vi "GetUIRef.vi"(8 "error in (no error)":errorcluster, 11 "Controller in":refnum<class "Controller.lvclass">) -> (0 "error out":errorcluster, 2 "VIRef":refnum<vi>, 3 "Controller out":refnum<class "Controller.lvclass">)   [LabVIEW 2020, in "UIHome.lvlib" / "Controller.lvclass"]
uses:
  Controller.lvclass
  Controller.lvclass/Controller.ctl
  iView/iView.lvclass
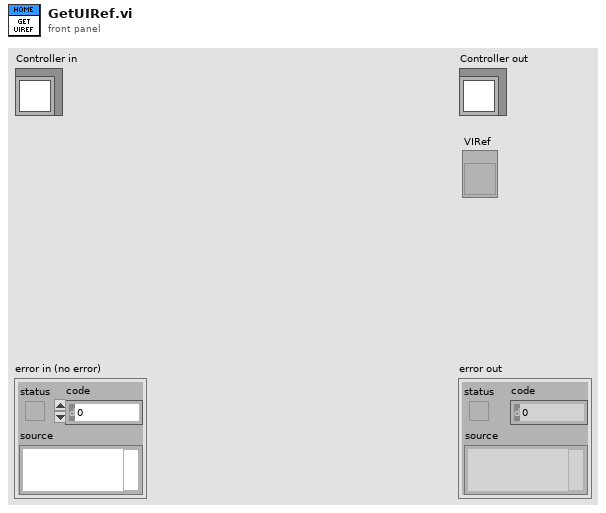
[diagram p1: front panel]
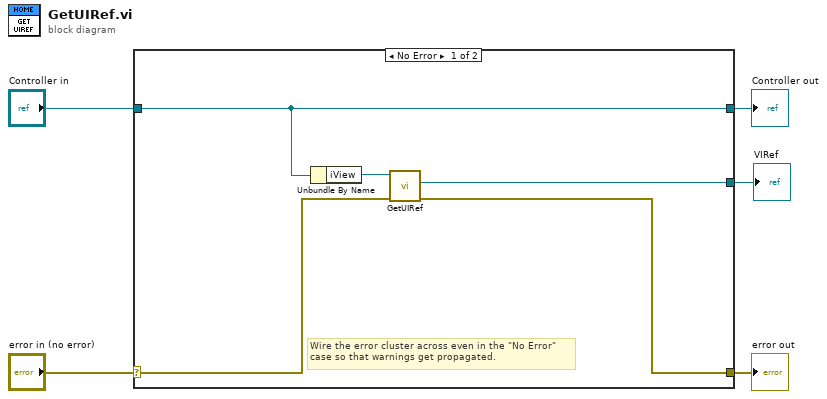
[diagram p0: block diagram]
diagram:
  n1 = case shown="No Error" "error in (no error)" {
    selector: "error in (no error)" -> [w7 w12]
    tunnel: [w6 w12] -> w4
    tunnel: [w10 w11] -> w2
    tunnel: "Controller in" -> [w10 w11]
    tunnel: [w8 _] -> w1
    frame No Error {
      # "Wire the error cluster across even in the \"No Error\"\ncase so that warnings get propagated."
      n2 = Unbundle By Name(w10) -> ("iView"=w9:refnum<class "iView.lvclass">)
      n3 = call-dynamic "GetUIRef.vi"("error in (no error)"=w7, "iView in"=w9) -> ("error out"=w6:errorcluster, "VIRef"=w8:refnum<vi>)  [unwired: 7 in, 1 out]
    }
    frame Error {
    }
  }
  "error out" <- w4
  "Controller out" <- w2
  "VIRef" <- w1
